vi "gyro-sweeper-V2.vi"() -> ()   [LabVIEW 2017]
uses:
  lorentzian.ctl
  circle corners.ctl
  peak -- parameters -- complex fit.ctl
  wavepacket.ctl
  filter method control.ctl
  cursor winow.ctl
  parameters -- scan monitor control.ctl
  freq scan type.ctl
  filename-pattern.ctl
  show-win- control.ctl
  PLL data source.ctl
  plot refs -- filter related.ctl
  cursor window action.ctl
  data source action.ctl
  publisher action.ctl
  file -- read-write control.ctl
  KM_file -- read-write control.ctl
  filename-action.ctl
  agregator -- action.ctl
  cursor action.ctl
  2Dwindow.ctl
  <vilib>/Analysis/baseanly.llb/A x B.vi
  <vilib>/Analysis/baseanly.llb/Complex A x B.vi
  line -- complex.vi
  Q -- check range -- i -- integer.vi
  Q - not nan -- real.vi
  linear interpolation - real.vi
  filter - complex - four.vi
  peak -- PM find lorenzian - V3.vi
  array -- sort 2D array -- Complex.vi/05c44075-957c-bc42-b6fa-2799d0bc0485.vi
  Q - not nan -- integer.vi
  tale of three indices.vi
  filter -- window span logic.vi
  linear interp iiii- complex - z-omega - divide.vi
  linear interpolation iiii- complex.vi
  containing bix.vi
  peak -- guess at omega -- dzdomega V2.vi
  <vilib>/Array/Sort 2D Array - Pop Stack.vi
  <vilib>/Array/Sort 2D Array - Push Stack.vi
  command stack.vi
  tale of three indices -- check state.vi
  peak -- z center from mult phase points.vi
  peak -- estimate for lorentzian.vi
  peak -- fake phase around center.vi
  peak -- get weights.vi
  peak -- four corner circle transformation logic.vi
  peak - fit phase around center - V2.vi
  circle center from three points.vi
  <vilib>/Utility/error.llb/Clear Errors.vi
  <vilib>/Analysis/Matrix/Numeric/Conversions/Array To Matrix.vi
  <vilib>/Analysis/Matrix/Numeric/Conversions/Array To Matrix - RA2.vi
  <vilib>/Analysis/baseanly.llb/Inverse Matrix.vi
  <vilib>/Analysis/baseanly.llb/Real Inverse Matrix.vi
  peak -- fit function -- minus arctan.vi
  <vilib>/gmath/NumericalOptimization/Nonlinear Curve Fit.vi
  <vilib>/gmath/NumericalOptimization/Nonlinear Curve Fit LM.vi
  KM_filter pipe - plot staff - more - V3.vi
panel:
  in  "all":enum32{"all"}(tab)
  in  "subtract bgnd !":bool
  out "Plot: circle sweep window":cluster{"all rows":dbl[], "all rows":dbl[]}[](graph)
  in  "sweeper panel":enum32{"circles sweep", "other"}(tab)
  in  "history length":i64=5
  out "fit is fine":bool=TRUE
  in  "gamma factor":dbl=1.6
  in  "Auto-update sweep window!":bool
  in  "scan type":T1
  in  "N":i64=257
  in  "sweep! :r":bool
  in  "delay-circle(msec)":i64
  out "scan progress":i32(slide)=256 min=0 max=257 scale=0.0..257.0
  out "circle frequency (Hz)":dbl=44934.75723893914 format="%#11_11f"
  out "circle gamma (Hz)":dbl=11.158120659005691 format="%#11_11f"
  out "circle phase (rad)":dbl=-1.4840328638382214 format="%#11_11f"
  out "circle Q":dbl=4027.0900998612533 format="%#11_11f"
  in  "beep!":bool
  in  "save data":enum32{"save/read"}(tab)
  in  "freqsweep name template":T2={"prefix"="lsco0.2", "group"="f"}
  in  "Save folder":path=path "/Users/arkady/Desktop/local_data/TaAs-quirk-Jan2018-losalamos"
  in  "freq sweep file name":string="f010_lsco0.2_012518.dat"
  in  "read from disk :l":bool
  in  "read file":path=path "/Users/arkady/Desktop/local_data/TaAs-quirk-Jan2018-losalamos/9w/f006_rucl3_012518.dat"
  in  "win":T3={"cen (Hz)"=44935.274309827895, "win (Hz)"=39.462177081403425, "left (Hz)"=44915.5432212872, "right (Hz)"=44955.005398368594}
  in  "PLL data source":T4=enum."MFLI"
  in  "Tab : everything":enum32{"Everything", "even more "}(tab)
  in  "Tab :  Fit controls":enum32{"complex plane", "complex plane 2"}(tab)
  in  "Plot: fragment - filter":cluster{dbl[], dbl[]}[](graph)=[{array[255 elements], array[255 elements]}, {array[255 elements], array[255 elements]}, {array[255 elements], array[255 elements]}, {array[255 elements], array[255 elements]}]
  in  "scale gauge: Plot: complex plane - filter":dbl(slide)=9.999999999999991e-05 min=0.0 max=0.3 step=1e-05 scale=0.0001..0.3 scale format="%#_5g"
  in  "Plot: complex plane - filter":cluster{dbl[], dbl[]}[](graph)=[{array[255 elements], array[255 elements]}, {array[255 elements], array[255 elements]}, {[-8.455997466784519e-05, -8.536551810596276e-05, -8.777896930838301e-05, -9.1790803485811e-05, -9.73851877615811e-05, -0.00010454004365678785, -0.00011322713422395566, -0.00012341217548537004, -0.00013505497173627495, -0.00014810957417895574, -0.00016252446226165164, -0.0001782427470066363, -0.00019520239552502235, -0.00021333647583223424, -0.00023257342099797256, -0.00025283731158819243, -0.00027404817528442526, -0.0002961223024979839, -0.0003189725767334659, -0.0003425088183977611, -0.0003666381406977065, -0.000391265316221823, -0.00041629315275940325, -0.00044162287687376416, -0.00046715452371587666, -0.000492787331539955, -0.000518420139364033, -0.0005439517862061456, -0.0005692815103205066, -0.0005943093468580867, -0.0006189365223822033, -0.0006430658446821486, -0.0006666020863464437, -0.0006894523605819259, -0.0007115264877954845, -0.0007327373514917173, -0.0007530012420819372, -0.0007722381872476754, -0.0007903722675548874, -0.0008073319160732736, -0.0008230502008182579, -0.000837465088900954, -0.0008505196913436348, -0.0008621624875945397, -0.0008723475288559541, -0.0008810346194231219, -0.0008881894753183286, -0.0008937838595940987, -0.0008977956937715266, -0.0009002091449739469, -0.0009010146884120644, -0.0009002091449739469, -0.0008977956937715266, -0.0008937838595940986, -0.0008881894753183286, -0.0008810346194231219, -0.000872347528855954, -0.0008621624875945397, -0.0008505196913436348, -0.000837465088900954, -0.0008230502008182579, -0.0008073319160732733, -0.0007903722675548873, -0.0007722381872476754, -0.0007530012420819371, -0.0007327373514917174, -0.0007115264877954843, -0.0006894523605819258, -0.0006666020863464435, -0.0006430658446821485, -0.0006189365223822033, -0.0005943093468580865, -0.0005692815103205065, -0.0005439517862061453, -0.0005184201393640329, -0.000492787331539955, -0.0004671545237158765, -0.00044162287687376416, -0.000416293152759403, -0.00039126531622182294, -0.00036663814069770655, -0.00034250881839776096, -0.00031897257673346594, -0.0002961223024979837, -0.0002740481752844252, -0.0002528373115881922, -0.0002325734209979724, -0.00021333647583223424, -0.0001952023955250222, -0.0001782427470066362, -0.00016252446226165153, -0.00014810957417895563, -0.00013505497173627495, -0.00012341217548536993, -0.0001132271342239556, -0.00010454004365678774, -9.738518776158104e-05, -9.1790803485811e-05, -8.777896930838301e-05, -8.536551810596276e-05], [0.004141207599747948, 0.004166840407572026, 0.004192372054414139, 0.0042177017785285, 0.00424272961506608, 0.0042673567905901965, 0.004291486112890142, 0.004315022354554437, 0.004337872628789919, 0.004359946756003478, 0.004381157619699711, 0.004401421510289931, 0.004420658455455669, 0.004438792535762881, 0.004455752184281267, 0.004471470469026252, 0.004485885357108948, 0.004498939959551629, 0.004510582755802533, 0.004520767797063948, 0.004529454887631116, 0.004536609743526323, 0.004542204127802092, 0.0045462159619795205, 0.00454862941318194, 0.004549434956620058, 0.00454862941318194, 0.0045462159619795205, 0.004542204127802092, 0.004536609743526323, 0.004529454887631116, 0.004520767797063948, 0.004510582755802533, 0.004498939959551629, 0.004485885357108948, 0.004471470469026252, 0.004455752184281267, 0.004438792535762881, 0.004420658455455669, 0.004401421510289931, 0.004381157619699711, 0.004359946756003478, 0.004337872628789919, 0.004315022354554437, 0.004291486112890142, 0.0042673567905901965, 0.00424272961506608, 0.0042177017785285, 0.004192372054414139, 0.004166840407572026, 0.004141207599747948, 0.0041155747919238705, 0.004090043145081758, 0.0040647134209673965, 0.0040396855844298165, 0.0040150584089057, 0.0039909290866057545, 0.00396739284494146, 0.003944542570705978, 0.003922468443492419, 0.003901257579796186, 0.003880993689205966, 0.003861756744040228, 0.003843622663733016, 0.0038266630152146296, 0.0038109447304696454, 0.003796529842386949, 0.0037834752399442686, 0.0037718324436933634, 0.0037616474024319492, 0.0037529603118647815, 0.0037458054559695747, 0.0037402110716938048, 0.0037361992375163767, 0.0037337857863139565, 0.0037329802428758387, 0.0037337857863139565, 0.0037361992375163767, 0.0037402110716938048, 0.0037458054559695747, 0.0037529603118647815, 0.0037616474024319492, 0.0037718324436933634, 0.0037834752399442686, 0.003796529842386949, 0.0038109447304696454, 0.00382666301521463, 0.003843622663733016, 0.003861756744040228, 0.0038809936892059663, 0.0039012575797961863, 0.003922468443492419, 0.003944542570705978, 0.00396739284494146, 0.0039909290866057545, 0.0040150584089057, 0.0040396855844298165, 0.0040647134209673965, 0.004090043145081758, 0.0041155747919238705]}, {[0.00016018653422290237, -9.655871916433519e-05, 0.00023322284291397248], [-0.00028197255148921553, -1.017876794960279e-06, -0.00018735204694998037]}, {[0.00016865843187043812, 0.00017215317328655273, 0.00017564791470266734, 0.00017914265611878197, 0.00018263739753489658, 0.0001861321389510112, 0.0001896268803671258, 0.0001931216217832404, 0.00019661636319935505, 0.00020011110461546966, 0.00020360584603158427, 0.00020710058744769888, 0.0002105953288638135, 0.00021409007027992812, 0.00021758481169604273, 0.00022107955311215734, 0.00022457429452827195, 0.0002280690359443866, 0.00023156377736050117, 0.0002350585187766158], [-0.00027606938786554, -0.00027143787714636365, -0.00026680636642718733, -0.00026217485570801096, -0.00025754334498883464, -0.00025291183426965827, -0.00024828032355048195, -0.00024364881283130558, -0.00023901730211212924, -0.0002343857913929529, -0.00022975428067377655, -0.0002251227699546002, -0.00022049125923542386, -0.00021585974851624751, -0.00021122823779707114, -0.00020659672707789482, -0.00020196521635871845, -0.00019733370563954213, -0.00019270219492036576, -0.00018807068420118942]}, {[-9.655871916433519e-05, -9.088660415427566e-05, -8.521448914421613e-05, -7.95423741341566e-05, -7.387025912409707e-05, -6.819814411403754e-05, -6.252602910397802e-05, -5.685391409391849e-05, -5.118179908385896e-05, -4.550968407379943e-05, -3.98375690637399e-05, -3.416545405368038e-05, -2.8493339043620856e-05, -2.282122403356132e-05, -1.7149109023501796e-05, -1.147699401344226e-05, -5.804879003382736e-06, -1.3276399332321333e-07, 5.539351016736323e-06, 1.1211466026795846e-05], [-1.017876794960279e-06, -1.017876794960279e-06, -1.017876794960279e-06, -1.017876794960279e-06, -1.017876794960279e-06, -1.017876794960279e-06, -1.017876794960279e-06, -1.017876794960279e-06, -1.017876794960279e-06, -1.017876794960279e-06, -1.017876794960279e-06, -1.017876794960279e-06, -1.017876794960279e-06, -1.017876794960279e-06, -1.017876794960279e-06, -1.017876794960279e-06, -1.017876794960279e-06, -1.017876794960279e-06, -1.017876794960279e-06, -1.017876794960279e-06]}]
  out "Plot: dz/domega":cluster{"omega out":dbl[], dbl[]}(graph)
  out "Plot: win omega":T5(graph)
  out "Plot: phase":cluster{"omega out":dbl[], dbl[]}(graph)
  out "Plot: phase around center":cluster{dbl[], dbl[]}[](graph)
  out "Plot: fragment":cluster{dbl[], dbl[]}[](graph)
  out "Plot: complex plane":cluster{dbl[], dbl[]}[](graph)=[{array[255 elements], array[255 elements]}, {[-0.00010617557464667055, -0.00010929113388811687, -0.00011858867738207354, -0.00013392157731355743, -0.00015504802469121866, -0.0001816348428195835, -0.0002132627416945725, -0.000249432930457336, -0.0002895749836240618, -0.00033305583703661034, -0.0003791897716624629, -0.00042724922779349337, -0.0004764762790971875, -0.0005260945855676712, -0.0005753216368713655, -0.0006233810930023958, -0.0006695150276282485, -0.0007129958810407971, -0.0007531379342075228, -0.0007893081229702864, -0.0008209360218452751, -0.0008475228399736401, -0.0008686492873513014, -0.0008839821872827852, -0.0008932797307767419, -0.0008963952900181882, -0.0008932797307767419, -0.0008839821872827852, -0.0008686492873513013, -0.0008475228399736401, -0.0008209360218452751, -0.0007893081229702863, -0.0007531379342075226, -0.0007129958810407969, -0.0006695150276282483, -0.0006233810930023958, -0.0005753216368713655, -0.0005260945855676711, -0.00047647627909718735, -0.0004272492277934931, -0.00037918977166246303, -0.00033305583703661034, -0.00028957498362406167, -0.00024943293045733586, -0.00021326274169457238, -0.0001816348428195834, -0.00015504802469121866, -0.00013392157731355737, -0.00011858867738207348, -0.00010929113388811687], [0.004141386571247566, 0.004190906967324454, 0.0042396463971731595, 0.004286836210869443, 0.004331732196861486, 0.004373626318630633, 0.004411857880850249, 0.0044458239489457005, 0.004474988857732779, 0.0044988926591776396, 0.004517158376052058, 0.004529497947089514, 0.004535716769883444, 0.004535716769883444, 0.004529497947089514, 0.004517158376052058, 0.0044988926591776396, 0.004474988857732779, 0.0044458239489457005, 0.004411857880850249, 0.004373626318630633, 0.004331732196861486, 0.004286836210869443, 0.0042396463971731595, 0.004190906967324454, 0.004141386571247566, 0.004091866175170678, 0.004043126745321973, 0.003995936931625689, 0.003951040945633646, 0.003909146823864499, 0.0038709152616448837, 0.0038369491935494313, 0.003807784284762353, 0.0037838804833174922, 0.0037656147664430744, 0.0037532751954056187, 0.0037470563726116884, 0.0037470563726116884, 0.0037532751954056187, 0.0037656147664430744, 0.0037838804833174927, 0.003807784284762353, 0.0038369491935494318, 0.003870915261644884, 0.0039091468238645, 0.003951040945633646, 0.003995936931625689, 0.004043126745321973, 0.004091866175170678]}, {[-0.00010766181539318114, -0.00014702417708710596, -0.00018638653878103078, -0.00022574890047495562, -0.0002651112621688804, -0.00030447362386280526, -0.0003438359855567301, -0.0003831983472506549, -0.00042256070894457974, -0.0004619230706385046, -0.0005012854323324294, -0.0005406477940263542, -0.0005800101557202791, -0.0006193725174142039, -0.0006587348791081286, -0.0006980972408020535, -0.0007374596024959783, -0.0007768219641899032, -0.000816184325883828, -0.0008555466875777528], [0.004175624676161894, 0.004172200865670462, 0.004168777055179028, 0.004165353244687596, 0.0041619294341961625, 0.00415850562370473, 0.004155081813213298, 0.004151658002721864, 0.004148234192230432, 0.0041448103817389986, 0.004141386571247566, 0.004137962760756134, 0.0041345389502647, 0.004131115139773268, 0.004127691329281835, 0.004124267518790402, 0.00412084370829897, 0.004117419897807536, 0.004113996087316104, 0.004110572276824671]}, {[-0.0004670473274181016, -0.00047047113790953435, -0.0004738949484009671, -0.0004773187588923999, -0.0004807425693838327, -0.0004841663798752655, -0.00048759019036669825, -0.0004910140008581311, -0.0004944378113495638, -0.0004978616218409966, -0.0005012854323324294, -0.0005047092428238621, -0.0005081330533152949, -0.0005115568638067277, -0.0005149806742981604, -0.0005184044847895932, -0.000521828295281026, -0.0005252521057724587, -0.0005286759162638915, -0.0005320997267553243], [0.0037477629543083172, 0.0037871253160022423, 0.003826487677696167, 0.003865850039390092, 0.0039052124010840166, 0.003944574762777942, 0.003983937124471867, 0.004023299486165791, 0.004062661847859716, 0.004102024209553641, 0.004141386571247566, 0.004180748932941491, 0.004220111294635415, 0.0042594736563293404, 0.0042988360180232655, 0.0043381983797171906, 0.004377560741411115, 0.00441692310310504, 0.004456285464798965, 0.00449564782649289]}, {[-0.1345621971793873, -0.13512978580258067, -0.13561317033829676, -0.13601204868693562, -0.13632617156251337, -0.13655534264845795, -0.13669941872030045, -0.13675830973518588, -0.1367319788881469, -0.1366204426351058, -0.1364237706825901, -0.1361420859441681, -0.1357755644636322, -0.13532443530497684, -0.13478898040924134, -0.1341695344183057, -0.13346648446575046, -0.13268026993491067, -0.13181138218427568, -0.1308603642404062], [0.028525297489512894, 0.02516387834181004, 0.021789321345350735, 0.01840373548841113, 0.015009236651946362, 0.01160794628723345, 0.008201990090033556, 0.004793496672101276, 0.0013845962308715039, -0.00202258078184437, -0.00542590499132186, -0.008823249430713024, -0.01221249087033164, -0.015591511144602398, -0.0189581984758458, -0.022310448794070212, -0.02564616705194721, -0.028963268534148004, -0.0322596801602224, -0.03553334178020699]}, {[-0.14932045372175862, -0.14995047709350323, -0.15048703392814808, -0.15092978889513722, -0.15127846528702854, -0.15153284519242702, -0.15169276963217218, -0.151758138658695, -0.15172891141848174, -0.15160510617760614, -0.15138680031031368, -0.1510741302506653, -0.15066729140727042, -0.15016653804116298, -0.14957218310689657, -0.14888459805695803, -0.1481042126096217, -0.1472315144803895, -0.1462670490771847, -0.1452114191594896], [0.031207435410939594, 0.027476260156989427, 0.023730501890919596, 0.019972501589716637, 0.016204607881240743, 0.012429175576409409, 0.008648564197517528, 0.004865136503612697, 0.0010812570138476487, -0.002700709470266971, -0.0064783993427869856, -0.01024945167051118, -0.014011509668487843, -0.017762222172928385, -0.02149924511060856, -0.02522024296383766, -0.028922890230081127, -0.03260487287532401, -0.03626388978026658, -0.03989765417844949]}, {array[255 elements], array[255 elements]}]
  in  "scale gauge: Plot: complex plane":dbl(slide)=9.999999999999991e-05 min=0.0 max=0.3 step=1e-05 scale=0.0001..1.0 scale format="%#_2g"
  out "window width (kHz)":dbl=76.27809365793496
  out "window center (kHz)":dbl=3399.029286744401
  out "# of points in window":dbl=953.475933538175
  in  "use fast fit!":bool
  out "lorentzian":T6={"Amplitude"=0.004408683465620264, "omega(0)"=44934.75723893914, "Gamma"=11.158120659005691, "phase"=-1.4840328638382214, "Q"=4027.0900998612533, "Norm  Ampl"=nan, "z (inf)"=-0.00010766181539318109+0.004175624676161894i, "4corners"={"z (-pi/2)"=-0.00046704732741810164+0.0037477629543083177i, "z(inf)"=-0.00010766181539318109+0.004175624676161894i, "z (pi/2)"=-0.0005355235372467572+0.004535010188186815i, "z center"=-0.0005012854323324294+0.004141386571247566i, "z(0)"=-0.0008949090492716776+0.004107148466333238i, "radius"=0.00039510985768575883}} {"z (inf)" format="%#9_9f"; "Q" format="%#9_9f"; "phase" format="%#9_9f"; "Gamma" format="%#9_9f"; "omega(0)" format="%#9_9f"}
  in  "plot staff!":enum16{"plot", "do not plot", "a"}(ring)
  in  "fit!":bool=TRUE
  in  "scan monitor control":T8={"gamma acc. frac. - min "=0.3, "gamma acc frac.. - max"=3.0, "peak acc. fraction (af)"=5.0, "min peak acc. window (kHz)"=0.5, "use"=enum."fraction", "abs gamma min(kHz)"=0.005, "abs gamma max(kHz)"=5.0, "# points"=5, "gamma-factor (fa)"=3.0, "interpolate"=enum."line", "init"=TRUE, "Unique strike parameters"=TRUE, "max peak acc. window (kHz)"=10.0, "spacing factor"=1.5, "iterate #"=1, "overwrite ctl?"=FALSE, "write _m files?"=FALSE, "max slope (kHz/sweep)"=0.5, "funnel state"=enum."funnel open"}
  in  "parameters: complex fit":T9={"main VI path"=path "", "scale factor"=3.0, "# of grid points"=200, "parameters: wavepacket"={"R"=0.5, "wave number"=22.0, "delta k"=7.0, "radii vector"=[], "radial section"=[], "wave vector"=22.0, "wavepacket is"=TRUE}, "span"=0.27789, "interference ?"=enum."cp z center", "filter method"=enum."three"} {"span" min=0.0 max=0.5 step=1e-05 scale=0.0001..0.5 scale format="%#_5f"; "parameters: wavepacket"."delta k" format="%#_3f"; "parameters: wavepacket"."wave number" format="%#_3f"; "parameters: wavepacket"."R" format="%#_3f"}
  in  "cursor bracket: circle window":T12={"left"=44915.5432212872, "right "=44955.005398368594, "center"=44935.274309827895, "window"=39.462177081403425, "cursors"=[0, 1, 2], "relative"=0, "absolute"=0, "fixed vertical offset"=0.0, "vertical offset"=0.0, "skew"=0.0, "default window frac"=0.1, "kind"=enum."symmetric", "skew.left"=0.5, "skew.right"=0.5, "Plot ref"=refnum, "wing order"=enum."forw"}
  in  "cursor bracket: fit boundaries":T12={"left"=45113.93683640631, "right "=45686.175933405, "center"=45400.056384905656, "window"=572.2390969986809, "cursors"=[3, 4, 5], "relative"=0, "absolute"=0, "fixed vertical offset"=0.0, "vertical offset"=0.0, "skew"=0.0, "default window frac"=0.1, "kind"=enum."symmetric", "skew.left"=0.5, "skew.right"=0.5, "Plot ref"=refnum, "wing order"=enum."forw"}
  # "three strikes"
  # "search window"
  # "linear extrapolation"
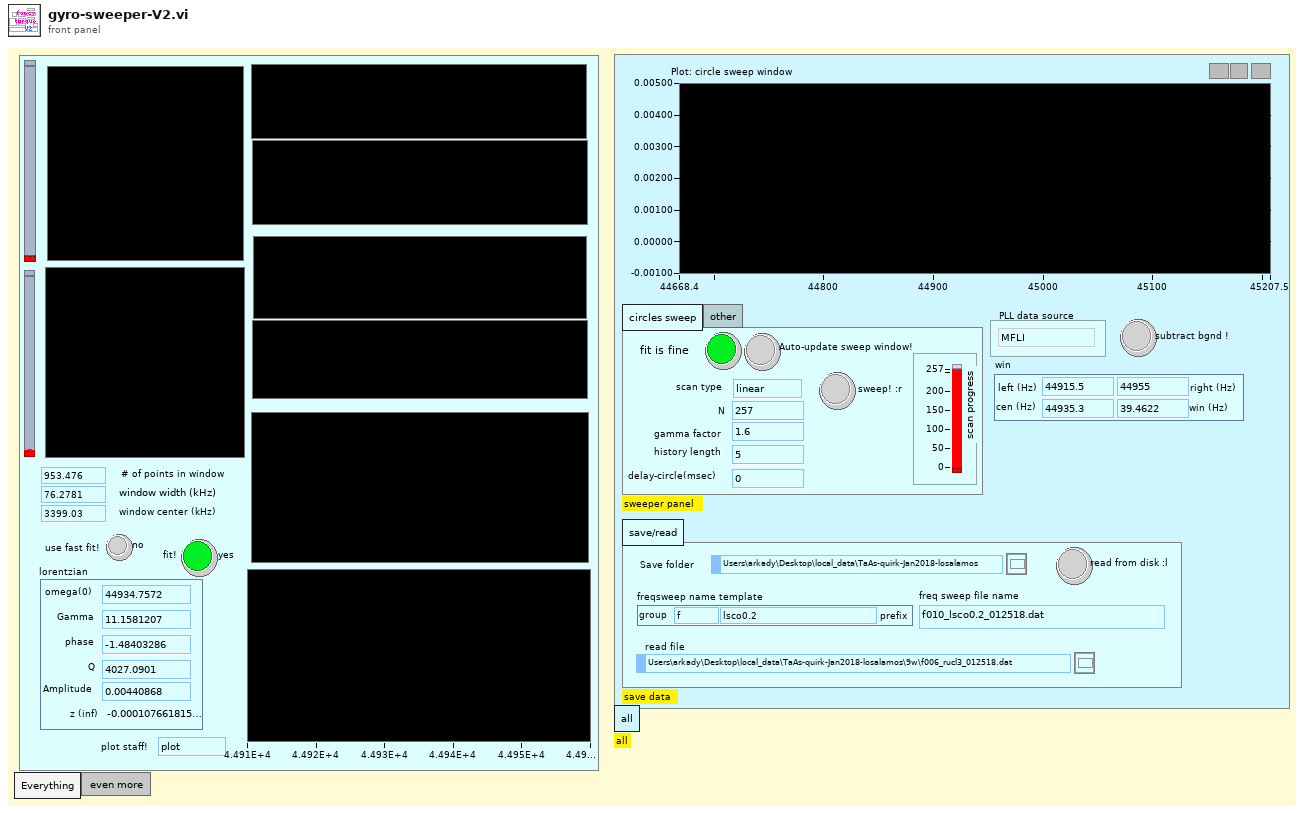
[diagram p1: front panel]
types:
  T1 = typedef "freq scan type.ctl" = enum16{"linear", "arctan"}
  T2 = typedef "filename-pattern.ctl" = cluster{"prefix":string, "group":string}
  T3 = typedef "show-win- control.ctl" = cluster{"cen (Hz)":dbl, "win (Hz)":dbl, "left (Hz)":dbl, "right (Hz)":dbl}
  T4 = typedef "PLL data source.ctl" = enum16{"meta", "MFLI"}
  T5 = cluster{"omega out":dbl[], "win omega out":dbl[]}
  T6 = typedef "lorentzian.ctl" = cluster{"Amplitude":dbl, "omega(0)":dbl, "Gamma":dbl, "phase":dbl, "Q":dbl, "Norm  Ampl":dbl, "z (inf)":cdb, "4corners":T7}
  T7 = typedef "circle corners.ctl" = cluster{"z (-pi/2)":cdb, "z(inf)":cdb, "z (pi/2)":cdb, "z center":cdb, "z(0)":cdb, "radius":dbl}
  T8 = typedef "parameters -- scan monitor control.ctl" = cluster{"gamma acc. frac. - min ":dbl, "gamma acc frac.. - max":dbl, "peak acc. fraction (af)":dbl, "min peak acc. window (kHz)":dbl, "use":enum16{"window", "fraction"}, "abs gamma min(kHz)":dbl, "abs gamma max(kHz)":dbl, "# points":i32, "gamma-factor (fa)":dbl, "interpolate":enum16{"line", "last"}, "init":bool, "Unique strike parameters":bool, "max peak acc. window (kHz)":dbl, "spacing factor":dbl, "iterate #":i32, "overwrite ctl?":bool, "write _m files?":bool, "max slope (kHz/sweep)":dbl, "funnel state":enum16{"funnel open", "funnel closed"}}
  T9 = typedef "peak -- parameters -- complex fit.ctl" = cluster{"main VI path":path, "scale factor":dbl, "# of grid points":i32, "parameters: wavepacket":T10, "span":dbl, "interference ?":enum16{"cp z center", "pm zcenter", "fancy"}, "filter method":T11}
  T10 = typedef "wavepacket.ctl" = cluster{"R":dbl, "wave number":dbl, "delta k":dbl, "radii vector":dbl[], "radial section":cdb[], "wave vector":dbl, "wavepacket is":bool}
  T11 = typedef "filter method control.ctl" = enum16{"four", "five", "one", "two", "three", "zero", "minus one", "minus two"}
  T12 = typedef "cursor winow.ctl" = cluster{"left":dbl, "right ":dbl, "center":dbl, "window":dbl, "cursors":i32[], "relative":i32, "absolute":i32, "fixed vertical offset":dbl, "vertical offset":dbl, "skew":dbl, "default window frac":dbl, "kind":enum16{"symmetric", "skewed", "fancy"}, "skew.left":dbl, "skew.right":dbl, "Plot ref":refnum<vi>, "wing order":enum16{"forw", "back"}}
  T13 = typedef "data source action.ctl" = enum16{"set", "get", "init"}
  T14 = typedef "cursor window action.ctl" = enum16{"balance", "h. offset change", "cursor moves", "change center", "change window", "init", "check", "reset", "set y to middle", "idle", "-write all Y", "-write left.X", "-write center.X", "-write right.X", "-write all X", "-change center", "-change window", "-change skew", "-read cursor 2", "-read cursor 1", "-read cursor 0", "-read all cursors", "-reset", "-read plot scale", "-set y to middle", "-Q: center.Y is visible", "-Q: window is visible", "-parse center.Y", "-right left from center", "-left move", "-right move", "-set center.Y", "-empty", "-set cursors to default", "-check", "-write center.Y", "-copy cursor 1", "-copy cursor 0", "-copy cursor 2", "move right", "move left", "shrink", "broaden", "skew up", "skew down", "-write plot scale", "zoom X", "change cen&win", "zoom to all data", "color--red", "color--green", "color--yellow", "read", "zoom out", "zoom in", "slide right", "slide left", "set range aspect ratio to 1"}
  T15 = typedef "plot refs -- filter related.ctl" = cluster{"Plot: complex plane - filter":refnum<vi>, "Plot: dz/domega":refnum<vi>, "Plot: fragment filter":refnum<vi>, "Plot: win omega":refnum<vi>, "Plot: phase":refnum<vi>, "Plot: phase around center":refnum<vi>, "Plot: complex plane":refnum<vi>, "Plot: fragment":refnum<vi>}
  T16 = typedef "publisher action.ctl" = enum16{"set", "get"}
  T17 = typedef "file -- read-write control.ctl" = enum16{"read", "write all", "append one line"}
  T18 = typedef "filename-action.ctl" = enum16{"rewrite", "parse", "force pattern", "uniquenum"}
  T19 = typedef "KM_file -- read-write control.ctl" = enum16{"read", "write all", "append one line"}
  T20 = typedef "agregator -- action.ctl" = enum16{"append", "interpolate", "empty!", "force", "init", "scale", "read last"}
  T21 = typedef "interpolation state - real.ctl" = cluster{"requested size":i32, "Array":dbl[], "actual number of elements":i32}
  T22 = typedef "2Dwindow.ctl" = cluster{"window y":dbl, "center x":dbl, "center y":dbl, "window x":dbl}
  T23 = typedef "cursor action.ctl" = enum16{"range", "read", "write", "check", "zoom out", "smart zoom out", "zoom to aspect ratio 1", "zoom to win", "zoom out 20%", "zoom in 20%"}
  T24 = typedef "eventvkey.ctl" = enum16{"ASCII", "Enter", "Return", "Shift", "Ctrl", "Alt", "Cmd", "Opt", "Caps", "NumLock", "Clear", "Break", "Up", "Down", "Left", "Right", "Insert", "Delete", "Home", "End", "PageUp", "PageDown", "Escape", "Help", "Pause", "ScrollLock", "F1", "F2", "F3", "F4", "F5", "F6", "F7", "F8", "F9", "F10", "F11", "F12", "F13", "F14", "F15", "F16", "F17", "F18", "F19", "F20", "F21", "F22", "F23", "F24", "Play", "VolumeUp", "VolumeDown", "Mute", "Two Byte Char"}
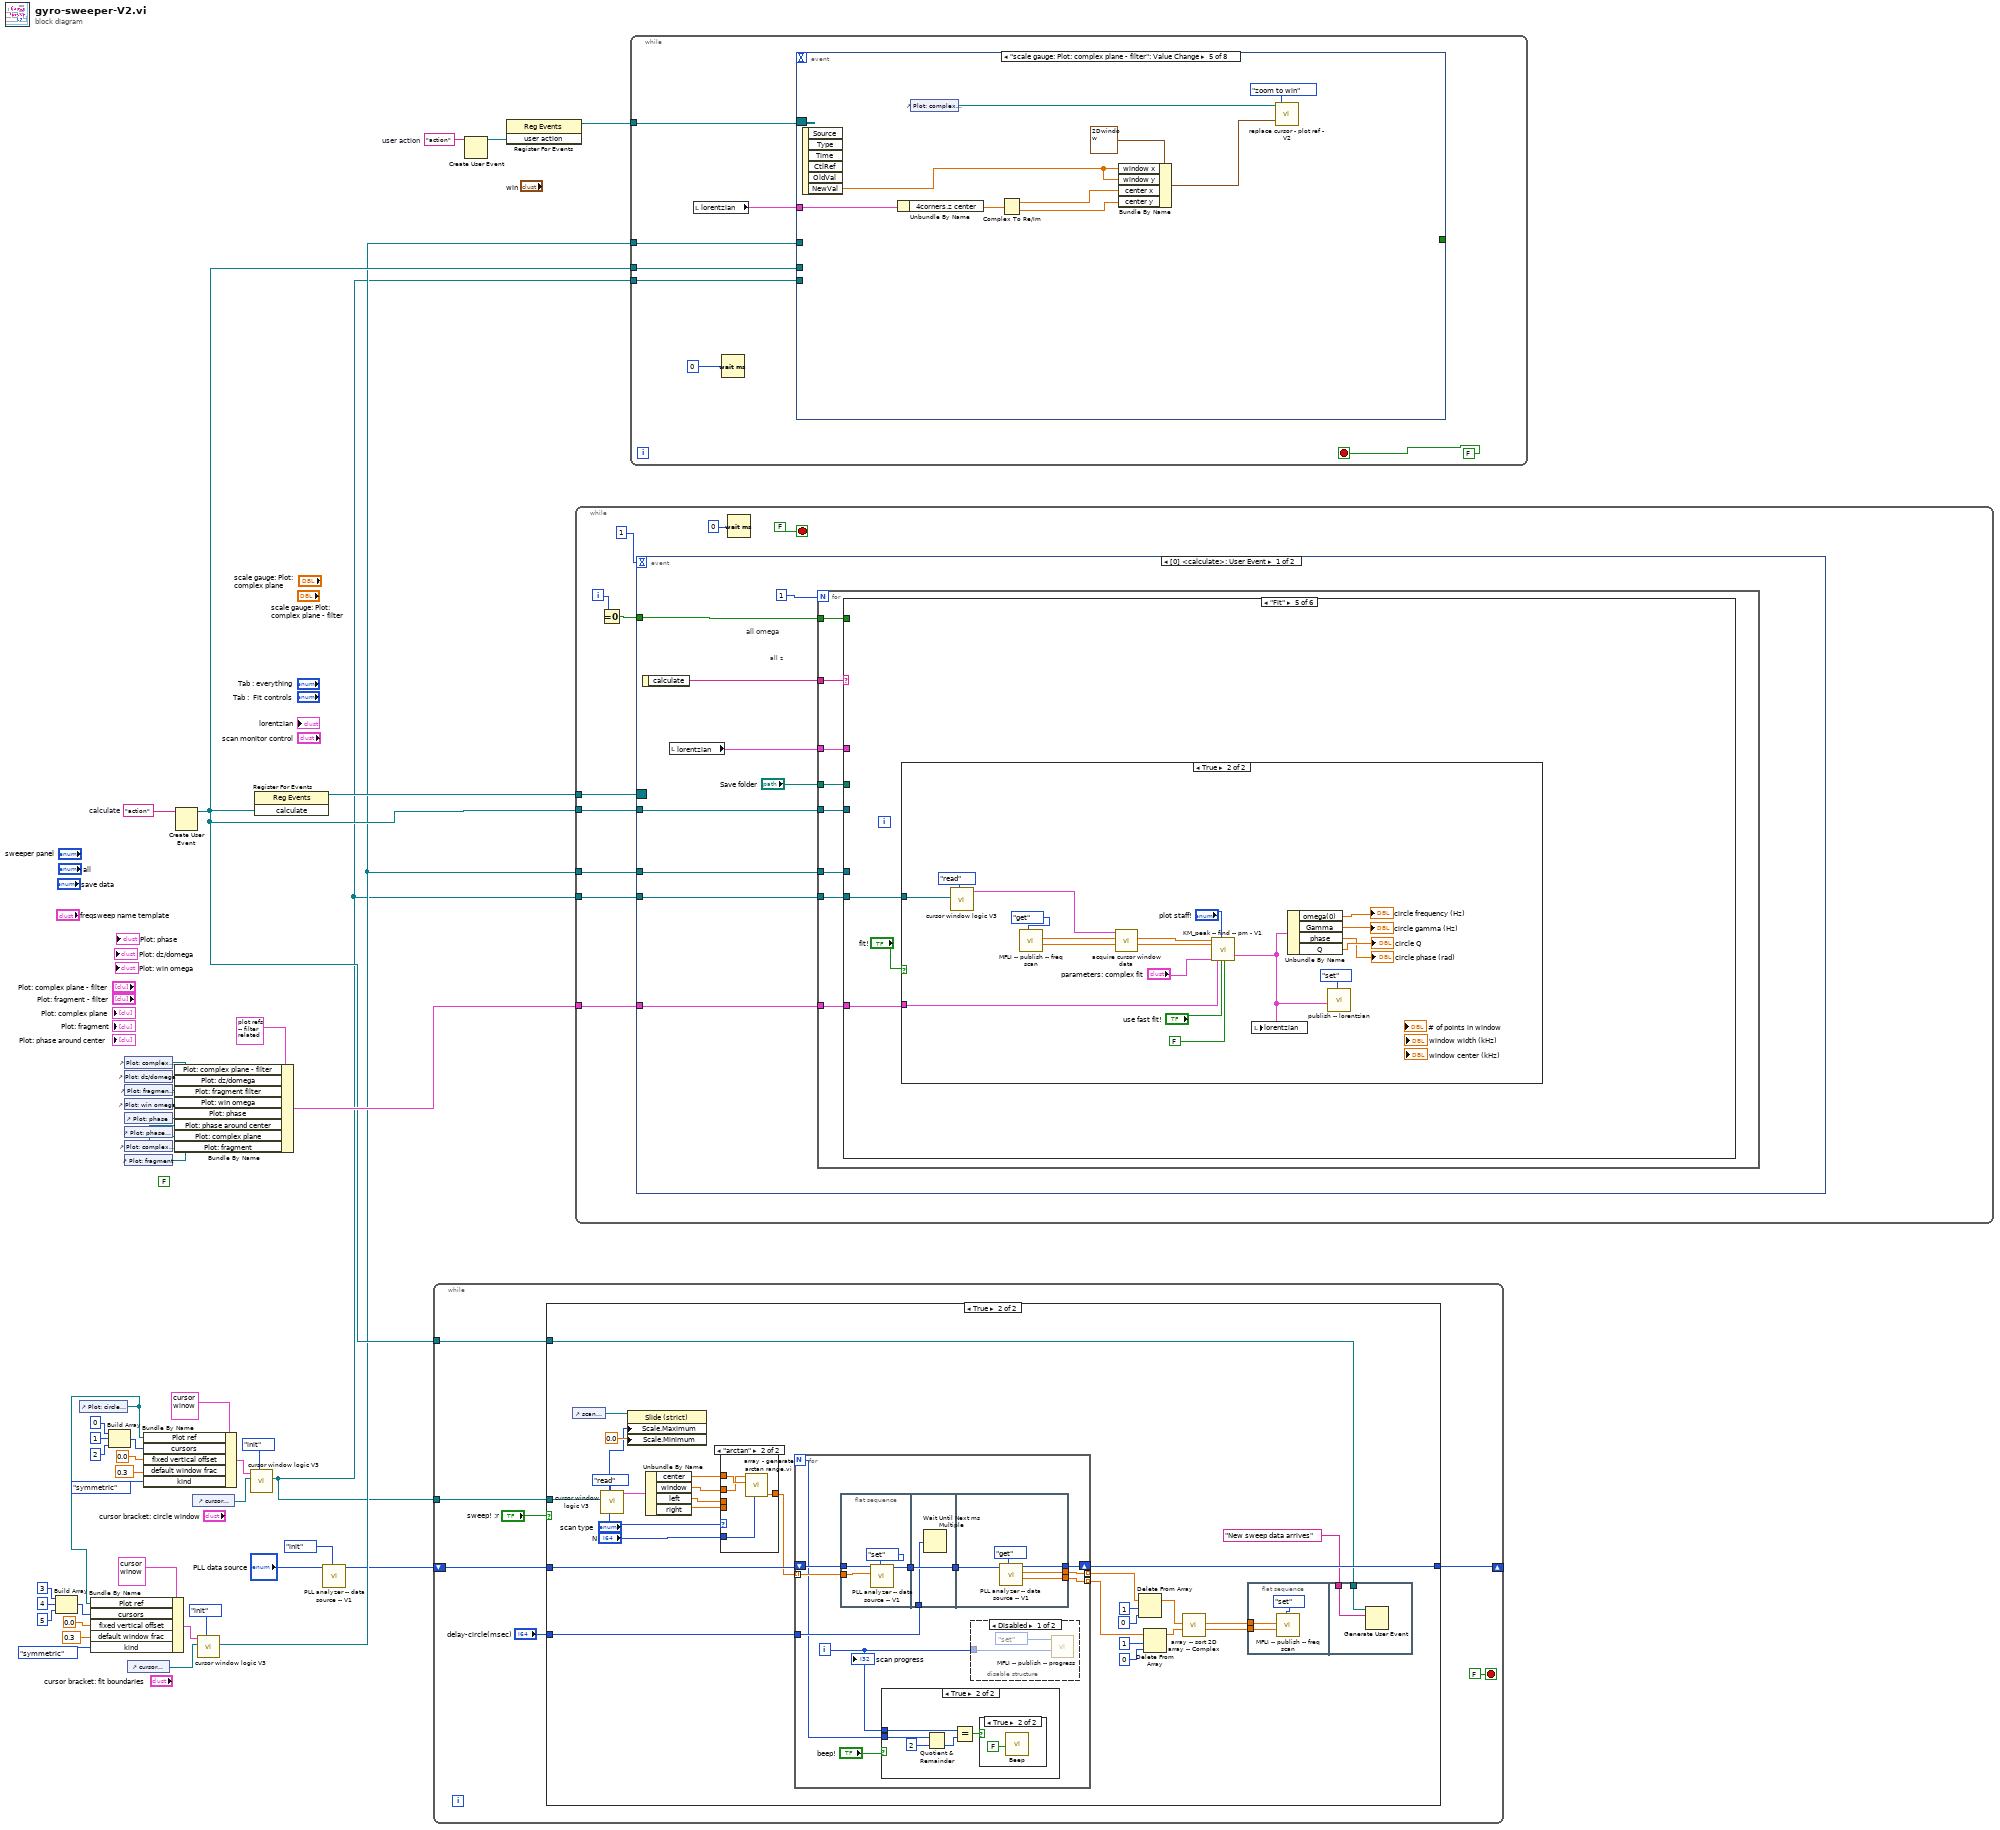
[diagram p0: block diagram]
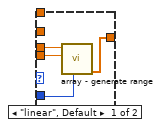
[diagram p6: hidden frame]
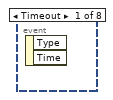
[diagram p7: hidden frame]
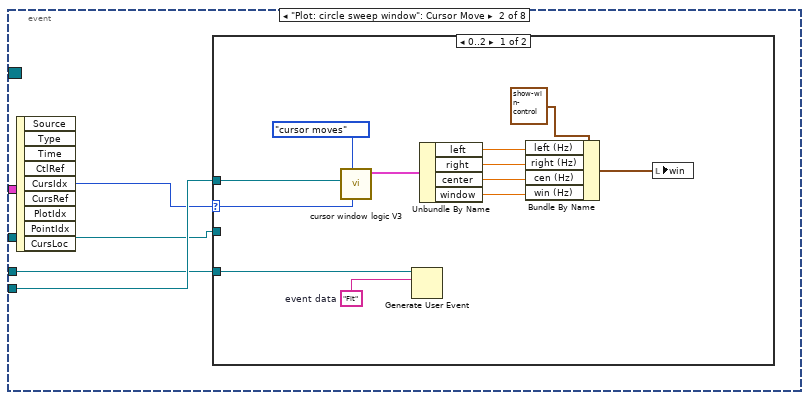
[diagram p8: hidden frame]
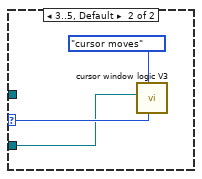
[diagram p9: hidden frame]
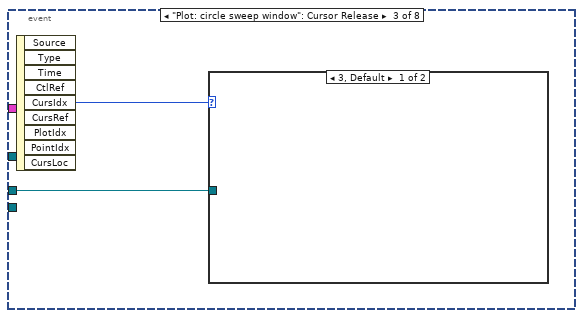
[diagram p10: hidden frame]
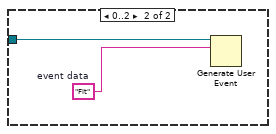
[diagram p11: hidden frame]
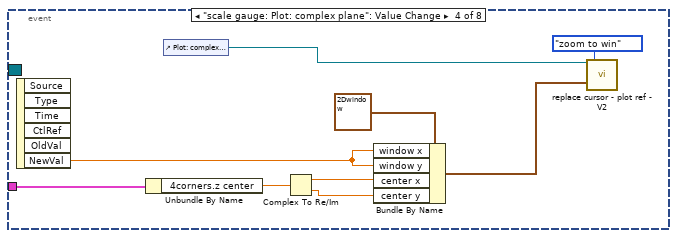
[diagram p12: hidden frame]
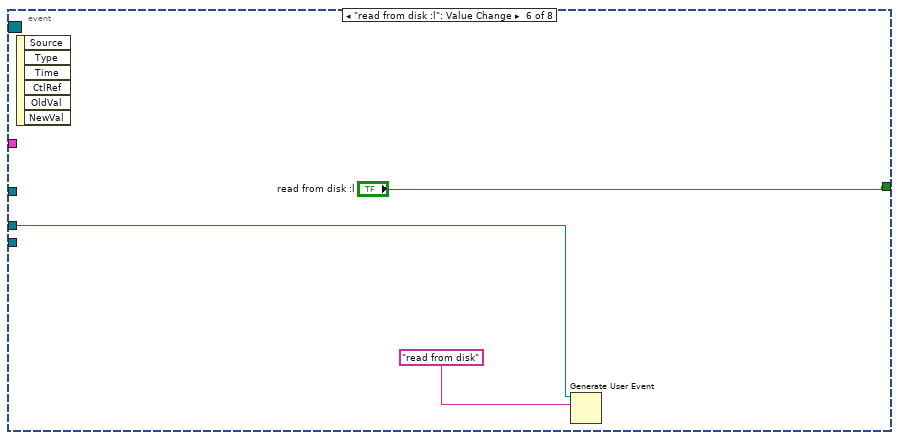
[diagram p13: hidden frame]
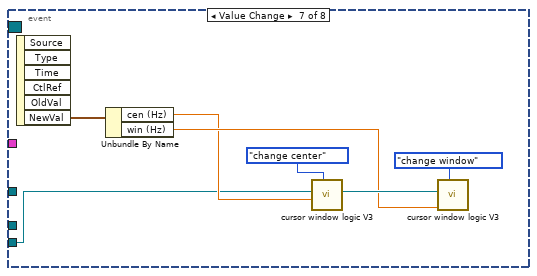
[diagram p14: hidden frame]
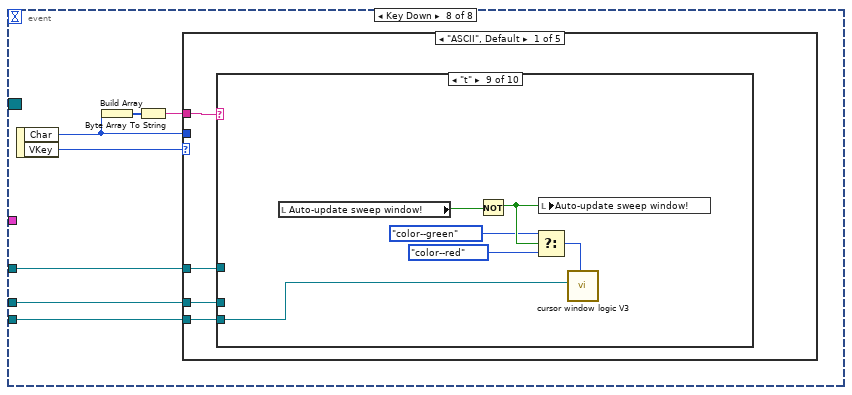
[diagram p15: hidden frame]
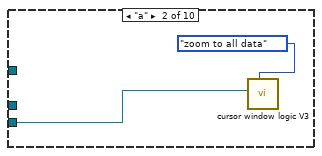
[diagram p17: hidden frame]
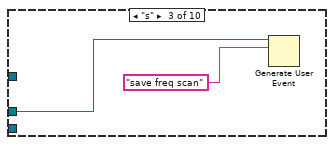
[diagram p18: hidden frame]
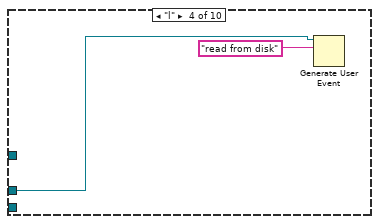
[diagram p19: hidden frame]
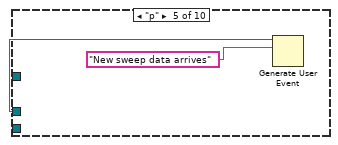
[diagram p20: hidden frame]
diagram:
  w41 = "action"  # user action
  w43 = "action"  # calculate
  (unwired) FALSE
  n1 = Build Array(3, 4, 5) -> (w17:i32[])
  n2 = control-ref of="Plot: circle sweep window"() -> (w6:refnum<vi>)
  n3 = Bundle By Name(cluster=T12 {"left"=0.0, "right "=0.0, "center"=0.0, "window"=0.0, "cursors"=[], "relative"=0, "absolute"=0, "fixed vertical offset"=0.0, "vertical offset"=0.0, "skew"=0.0, "default window frac"=0.0, "kind"=enum."symmetric", "skew.left"=0.0, "skew.right"=0.0, "Plot ref"=refnum, "wing order"=enum."forw"} ("cursor bracket: All, data window"), "Plot ref"=w6, "cursors"=w17, "fixed vertical offset"=0.0, "default window frac"=0.3 ("fixed vertical offset"), "kind"=enum16{"symmetric", "skewed", "fancy"}."symmetric") -> (w9:T12)
  n4 = Build Array(0, 1, 2) -> (w28:i32[])
  n5 = control-ref of="Plot: complex plane - filter"() -> (w38:refnum<vi>)
  n6 = control-ref of="Plot: dz/domega"() -> (w37:refnum<vi>)
  n7 = control-ref of="Plot: fragment - filter"() -> (w36:refnum<vi>)
  n8 = control-ref of="Plot: win omega"() -> (w35:refnum<vi>)
  n9 = control-ref of="Plot: phase"() -> (w34:refnum<vi>)
  n10 = control-ref of="Plot: phase around center"() -> (w32:refnum<vi>)
  n11 = control-ref of="Plot: complex plane"() -> (w31:refnum<vi>)
  n12 = control-ref of="Plot: fragment"() -> (w30:refnum<vi>)
  n13 = control-ref of="cursor bracket: fit boundaries"() -> (w7:refnum<vi>)
  n14 = Bundle By Name(cluster=T12 {"left"=0.0, "right "=0.0, "center"=0.0, "window"=0.0, "cursors"=[], "relative"=0, "absolute"=0, "fixed vertical offset"=0.0, "vertical offset"=0.0, "skew"=0.0, "default window frac"=0.0, "kind"=enum."symmetric", "skew.left"=0.0, "skew.right"=0.0, "Plot ref"=refnum, "wing order"=enum."forw"} ("cursor bracket: All, data window"), "Plot ref"=w6, "cursors"=w28, "fixed vertical offset"=0.0, "default window frac"=0.3 ("fixed vertical offset"), "kind"=enum16{"symmetric", "skewed", "fancy"}."symmetric") -> (w20:T12)
  n15 = Bundle By Name(cluster=T15 {"Plot: complex plane - filter"=refnum, "Plot: dz/domega"=refnum, "Plot: fragment filter"=refnum, "Plot: win omega"=refnum, "Plot: phase"=refnum, "Plot: phase around center"=refnum, "Plot: complex plane"=refnum, "Plot: fragment"=refnum} ("plots: filter related"), "Plot: complex plane - filter"=w38, "Plot: dz/domega"=w37, "Plot: fragment filter"=w36, "Plot: win omega"=w35, "Plot: phase"=w34, "Plot: phase around center"=w32, "Plot: complex plane"=w31, "Plot: fragment"=w30) -> (w33:T15)
  n16 = Create User Event(user event datatype=w43) -> (user event=w29:refnum<user-event>)  [unwired: 1 in, 1 out]
  n17 = control-ref of="cursor bracket: circle window"() -> (w19:refnum<vi>)
  n18 = call "cursor window logic V3.vi"("cursor window action"=cursor_window_action."init", "cursor window in"=w7, "cursor window init"=w9) -> ("cursor window out"=w5:refnum<vi>)  [unwired: 7 in, 1 out]
  n19 = call "cursor window logic V3.vi"("cursor window action"=cursor_window_action."init", "cursor window in"=w19, "cursor window init"=w20) -> ("cursor window out"=w4:refnum<vi>)  [unwired: 7 in, 1 out]
  n20 = register-events(w29) -> (reference out=w44:refnum<event-registration>)  [unwired: 2 in, 1 out]
  n21 = call "PLL analyzer -- data source -- V1.vi"("data source action"=data_source_action."init", "PLL data source"="PLL data source") -> ("PLL data source OUT"=w1:T4)  [unwired: 7 in, 2 out]
  n22 = while {
    tunnel: w29 -> [w51]
    tunnel: w4 -> [w49]
    shift-right: [w46] -> _
    shift-left: w1 -> [w45]
    stop <- FALSE stop-if-true
    n23 = case shown="True" "sweep! :r" {
      tunnel: w51 -> [_ w59]
      tunnel: w49 -> [_ w79]
      tunnel: "delay-circle(msec)" -> [_ w64]
      tunnel: [w52 w63] -> w46
      tunnel: w45 -> [w52 w62]
      frame False {
      }
      frame True {
        n24 = control-ref of="scan progress"() -> (w67:refnum<vi>)
        n25 = call "cursor window logic V3.vi"("cursor window action"=cursor_window_action."read", "cursor window in"=w79) -> ("cursor window out"=w69:T12)  [unwired: 8 in, 1 out]
        n26 = property class="Slide (strict)"(reference=w67, "Scale.Maximum"="N", "Scale.Minimum"=0.0 ("Data Entry Limits:Minimum")) -> ()  [unwired: 1 in, 2 out]
        n27 = Unbundle By Name(w69) -> ("center"=w73:dbl, "window"=w72:dbl, "left"=w71:dbl, "right"=w70:dbl)
        n28 = case shown="\"arctan\"" "scan type" {
          tunnel: [w113 w117] -> w53
          tunnel: w73 -> [_ w116]
          tunnel: w72 -> [_ w115]
          tunnel: w71 -> [w112 _]
          tunnel: w70 -> [w111 _]
          tunnel: "N" -> [w110 w114]
          frame "linear", Default {
            n29 = call "array - generate range.vi"("N"=w110, "freq max"=w111, "freq min"=w112) -> ("Array"=w113:dbl[])  [unwired: 7 in, 1 out]
          }
          frame "arctan" {
            n30 = call "array - generate arctan range.vi.vi"("N"=w114, "omega0"=w116, "gamma"=w115) -> ("Array"=w117:dbl[])  [unwired: 8 in]
          }
        }
        n31 = for {
          N -> [w81]
          tunnel: w53 -> [w90] mode=indexing
          tunnel: w64 -> [w87]
          shift-right: [w86] -> w63
          shift-left: w62 -> [w85]
          tunnel: [w84] -> w61 mode=indexing
          tunnel: [w83] -> w60 mode=indexing
          i -> [w82]
          n32 = flat-sequence {
            tunnel: w90 -> [w100]
            tunnel: [w101] -> w88
            tunnel: w85 -> [w99]
            tunnel: [w104] -> w89
            tunnel: w88 -> [w104]
            tunnel: w87 -> [w103]
            tunnel: w89 -> [w109]
            tunnel: [w108] -> w86
            tunnel: [w107] -> w84
            tunnel: [w106] -> w83
            frame #0 {
              n33 = call "PLL analyzer -- data source -- V1.vi"("data source action"=data_source_action."set", "Freq in (Hz)"=w100, "PLL data source"=w99) -> ("PLL data source OUT"=w101:T4)  [unwired: 6 in, 2 out]
            }
            frame #1 {
              n34 = Wait Until Next ms Multiple(millisecond multiple=w103) -> ()  [unwired: 1 out]
            }
            frame #2 {
              n35 = call "PLL analyzer -- data source -- V1.vi"("data source action"=data_source_action."get", "PLL data source"=w109) -> ("z out (V)"=w107:cdb, "Freq out (Hz)"=w106:dbl, "PLL data source OUT"=w108:T4)  [unwired: 7 in]
            }
          }
          n36 = case shown="True" "beep!" {
            tunnel: w82 -> [_ w94]
            tunnel: w81 -> [_ w93]
            frame False {
            }
            frame True {
              n37 = Quotient & Remainder(x=w93, y=2) -> (floor(x/y)=w96:i32)  [unwired: 1 out]
              n38 = Equal?(x=w94, y=w96) -> (x = y?=w95:bool)
              n39 = case shown="True" w95 {
                frame False {
                }
                frame True {
                  n40 = call <vilib>:"Beep.vi"("use system alert? (T) - ignored"=FALSE) -> ()  [unwired: 11 in]
                }
              }
            }
          }
          n41 = disable-structure shown="Disabled" {
            disable-tunnel: w82 -> [w91 _]
            frame Disabled {
              n42 = call "MFLI -- publish -- progress.vi"("publisher action"=publisher_action."set", "num"=w91) -> ()  [unwired: 9 in, 1 out]
            }
            frame Enabled {
            }
          }
          "scan progress" <- w82
        }
        n43 = Delete From Array(array=w60, length=1, index=0) -> (array with subset deleted=w57:dbl[])  [unwired: 1 out]
        n44 = Delete From Array(array=w61, length=1, index=0) -> (array with subset deleted=w56:cdb[])  [unwired: 1 out]
        n45 = call "array -- sort 2D array -- Complex.vi"("z In"=w56, "freq IN"=w57) -> ("z out"=w54:cdb[], "freq out"=w55:dbl[])  [unwired: 8 in]
        n46 = flat-sequence {
          tunnel: w54 -> [w119]
          tunnel: w55 -> [w118]
          tunnel: w59 -> [w122]
          tunnel: "New sweep data arrives" ("event data") -> [w121]
          frame #0 {
            n47 = call "MFLI -- publish -- freq scan.vi"("publisher action"=publisher_action."set", "Voltage IN (V)"=w119, "Freq IN (Hz)"=w118) -> ()  [unwired: 7 in, 2 out]
          }
          frame #1 {
            n48 = Generate User Event(user event=w122, event data cluster=w121) -> ()  [unwired: 2 in, 2 out]
          }
        }
      }
    }
  }
  n49 = Create User Event(user event datatype=w41) -> (user event=w40:refnum<user-event>)  [unwired: 1 in, 1 out]
  n50 = register-events(w40) -> (reference out=w42:refnum<event-registration>)  [unwired: 2 in, 1 out]
  n51 = while {
    tunnel: w44 -> [w132]
    tunnel: w29 -> [w130]
    tunnel: w33 -> [w126]
    tunnel: w4 -> [w124]
    tunnel: w5 -> [w123]
    i -> [w127]
    stop <- FALSE stop-if-true
    n52 = Equal To 0?(x=w127) -> (x = 0?=w125:bool)
    n53 = event shown="[0] <calculate>: User Event" {
      selector: w132 -> [_ _]
      dyn-events: _ -> [_ _]
      timeout: 1 -> [_ _]
      tunnel: w130 -> [w140 _]
      tunnel: w126 -> [w137 _]
      tunnel: w125 -> [w136 _]
      tunnel: w124 -> [w135 _]
      tunnel: w123 -> [w133 _]
      event User Event {
        # "all z"
        # "all omega"
        n54 = event-data() -> ("calculate"=w141:string)  [unwired: 1 in]
        n55 = local read "lorentzian"() -> (w134:T6)
        n56 = for {
          N: 1 -> [_]
          tunnel: w141 -> [w149]
          tunnel: w140 -> [w148]
          tunnel: "Save folder" -> [w147]
          tunnel: w137 -> [w146]
          tunnel: w136 -> [w145]
          tunnel: w135 -> [w144]
          tunnel: w134 -> [w143]
          tunnel: w133 -> [w142]
          n57 = case shown="\"Fit\"" w149 {
            tunnel: w148 -> [w160 w183 _ _ _ _]
            tunnel: w147 -> [_ _ w207 w229 _ _]
            tunnel: w146 -> [_ _ _ _ w251 _]
            tunnel: w145 -> [_ _ _ _ _ _]
            tunnel: w144 -> [_ _ _ w230 w250 _]
            tunnel: w143 -> [_ _ _ w228 _ _]
            tunnel: w142 -> [_ _ _ w221 _ _]
            frame "New sweep data arrives" {
              n58 = Generate User Event(user event=w160, event data cluster="Fit" ("event data")) -> (user event out=w151:refnum<user-event>)  [unwired: 2 in, 1 out]
              n59 = case shown="True" "Auto-update sweep window!" {
                tunnel: w151 -> [_ w181]
                frame False {
                }
                frame True {
                  n60 = Generate User Event(user event=w181, event data cluster="Update range" ("event data")) -> ()  [unwired: 2 in, 2 out]
                }
              }
              n61 = call "MFLI -- publish -- freq scan.vi"("publisher action"=publisher_action."get") -> ("Voltage out (V)"=w155:cdb[], "Freq out (Hz)"=w157:dbl[])  [unwired: 9 in]
              n62 = case shown="True" "subtract bgnd !" {
                tunnel: w157 -> [w172 w180]
                tunnel: [w166 w180] -> w156
                tunnel: w155 -> [w168 w179]
                tunnel: [w173 w179] -> w154
                frame True {
                  w165 = 10 ("length")
                  n63 = Delete From Array(array=w172, length=w165, index=0) -> (array with subset deleted=w171:dbl[])  [unwired: 1 out]
                  n64 = Delete From Array(array=w168, length=w165, index=0) -> (array with subset deleted=w167:cdb[])  [unwired: 1 out]
                  n65 = call "linear interp iiii- complex - z-omega.vi"("z"=w167, "omega"=w171) -> ("z out"=w174:cdb[], "omega out"=w166:dbl[], "intercept"=w176:cdb, "slope"=w177:cdb)  [unwired: 5 in, 5 out]
                  n66 = Multiply(x=w166, y=w177) -> (x*y=w178:cdb[])
                  n67 = Add(x=w178, y=w176) -> (x+y=w175:cdb[])
                  n68 = Subtract(x=w174, y=w175) -> (x-y=w173:cdb[])
                }
                frame False {
                }
              }
              n69 = Complex To Re/Im(x + iy=w154) -> (x=w163:dbl[], y=w162:dbl[])
              n70 = Bundle("Freq out (Hz)"=w156, w163) -> (w164:cluster{"Freq out (Hz)":dbl[], dbl[]})  [unwired: 1 in]
              n71 = Bundle("Freq out (Hz)"=w156, w162) -> (w161:cluster{"Freq out (Hz)":dbl[], dbl[]})  [unwired: 1 in]
              n72 = Build Array(w164, w161) -> (→"Plot: circle sweep window":cluster{"Freq out (Hz)":dbl[], dbl[]}[])
            }
            frame "read from disk" {
              n73 = call "file - read-write - list of lines.vi"("read/write control"=file_--_read-write_control."read", "file path"="read file") -> ("list of lines OUT"=w187:string[])  [unwired: 8 in, 1 out]
              n74 = for {
                tunnel: w187 -> [w197] mode=indexing
                tunnel: [w192] -> w188 mode=indexing
                tunnel: [w191] -> w189 mode=indexing
                w193 = 0.0
                n75 = Scan From String(format string="%f%f%f", input string=w197, default 1=w193, default 2=w193, default 3=w193) -> (output 1=w191:dbl, output 2=w195:dbl, output 3=w194:dbl)  [unwired: 2 in, 3 out]
                n76 = Re/Im To Complex(1:w194, 2:w195) -> (0:w192:cdb)
              }
              n77 = flat-sequence {
                tunnel: w183 -> [w201]
                tunnel: [w201] -> w190
                tunnel: w188 -> [w199]
                tunnel: w189 -> [w198]
                tunnel: w190 -> [w203]
                tunnel: "New sweep data arrives" ("event data") -> [w202]
                frame #0 {
                  n78 = call "MFLI -- publish -- freq scan.vi"("publisher action"=publisher_action."set", "Voltage IN (V)"=w199, "Freq IN (Hz)"=w198) -> ()  [unwired: 7 in, 2 out]
                }
                frame #1 {
                  n79 = Generate User Event(user event=w203, event data cluster=w202) -> ()  [unwired: 2 in, 2 out]
                }
              }
            }
            frame "save freq scan" {
              n80 = local read "freqsweep name template"() -> (w209:T2)
              n81 = call "MFLI -- publish -- freq scan.vi"("publisher action"=publisher_action."get") -> ("Voltage out (V)"=w204:cdb[], "Freq out (Hz)"=w205:dbl[])  [unwired: 9 in]
              n82 = call "filename-manage.vi"("filename pattern"=w209, "filename-action"=filename-action."uniquenum", "folder"=w207, "file name"="freq sweep file name") -> ("filename OUT"=w208:string)  [unwired: 7 in]
              n83 = call "KM_appendline -- freq sweep.vi"("freq"=w205, "Vout(V)"=w204, "Save frequency scan"=w207, "read/write control"=KM_file_--_read-write_control."append one line", "name or relative path"=w208) -> ()  [unwired: 15 in]
              n84 = local write "freq sweep file name"(w208) -> ()
            }
            frame "Update range" {
              n85 = call "cursor window logic V3.vi"("cursor window action"=cursor_window_action."read", "cursor window in"=w221) -> ("cursor window out"=w224:T12)  [unwired: 8 in, 1 out]
              n86 = Unbundle By Name(w224) -> ("left"=w223:dbl, "right"=w222:dbl, "window"=w216:dbl)
              n87 = Unbundle By Name(w228) -> ("omega(0)"=w219:dbl, "Gamma"=w226:dbl)
              n88 = Multiply(x=w216, y=3.0 ("lower")) -> (x*y=w217:dbl)
              n89 = Multiply(x=w216, y=0.0003 ("lower")) -> (x*y=w214:dbl)
              n90 = call "Q -- check range -- i -- real.vi"("upper"=w222, "lower"=w223, "number"=w219) -> ("in range?"=w227:bool)  [unwired: 6 in, 2 out]
              n91 = call "Q -- check range -- i -- real.vi"("upper"=w217, "lower"=w214, "number"=w226) -> ("in range?"=w225:bool)  [unwired: 6 in, 2 out]
              n92 = And(x=w227, y=w225) -> (x .and. y?=w220:bool)
              "fit is fine" <- w220
              n93 = case shown="True" w220 {
                tunnel: w226 -> [_ w238]
                tunnel: w219 -> [_ w233]
                tunnel: w230 -> [_ w239]
                tunnel: w229 -> [_ _]
                frame False {
                }
                frame True {
                  (unwired) agregator_--_action."append" ("aggregator action")
                  n94 = Compound Arithmetic op=MULTIPLY("gamma factor", w238, 2.0 ("value")) -> (w236:dbl)
                  n95 = for {
                    N: 1 -> [_]
                    tunnel: "history length" -> [w243]
                    tunnel: w233 -> [w248]
                    shift-right: [w244] -> _
                    shift-left: _ -> [w247]
                    tunnel: [w241] -> w232
                    n96 = call "aggregator - vii - real - atomic.vi"("aggregator action"=agregator_--_action."append", "requested size"=w243, "number"=w248, "state IN"=w247) -> ("state OUT"=w245:T21)  [unwired: 4 in, 3 out]
                    n97 = call "aggregator - vii - real - atomic.vi"("aggregator action"=agregator_--_action."interpolate", "requested size"=w243, "state IN"=w245) -> ("interp average"=w241:dbl, "state OUT"=w244:T21)  [unwired: 5 in, 2 out]
                  }
                  n98 = call "cursor window logic V3.vi"("cursor window action"=cursor_window_action."change cen&win", "window"=w236, "center"=w232, "cursor window in"=w239) -> ()  [unwired: 6 in, 2 out]
                }
              }
            }
            frame "Fit" {
              n99 = case shown="True" "fit!" {
                tunnel: w251 -> [_ w266]
                tunnel: w250 -> [_ w264]
                frame False {
                  (unwired) T6 {"Amplitude"=-1.0311345636926572, "omega(0)"=-1.0311345636926572, "Gamma"=-1.0311345636926572, "phase"=-1.0311345636926572, "Q"=-1.0311345636926572, "Norm  Ampl"=-1.0311345636926572, "z (inf)"=-1.0311345636926572+0.0i, "4corners"={"z (-pi/2)"=-1.0311345636926572+0.5736824521422934i, "z(inf)"=-0.5200164984937075+1.0975277942502903i, "z (pi/2)"=-1.0311345636926572+0.5736824521422934i, "z center"=-0.5136528600391839+0.580046090596817i, "z(0)"=-0.5200164984937075+1.0975277942502903i, "radius"=-1.0311345636926572}} ("pm lorentzian")
                }
                frame True {
                  n100 = call "cursor window logic V3.vi"("cursor window action"=cursor_window_action."read", "cursor window in"=w264) -> ("cursor window out"=w261:T12)  [unwired: 8 in, 1 out]
                  n101 = call "MFLI -- publish -- freq scan.vi"("publisher action"=publisher_action."get") -> ("Voltage out (V)"=w252:cdb[], "Freq out (Hz)"=w253:dbl[])  [unwired: 9 in]
                  n102 = call "acquire cursor window data.vi"("z in"=w252, "omega in"=w253, "cursor window"=w261) -> ("z out"=w262:cdb[], "omega  out"=w263:dbl[])  [unwired: 4 in, 3 out]
                  n103 = call "KM_peak -- find -- pm - V1.vi"("omega in"=w263, "z in"=w262, "parameters: complex fit"="parameters: complex fit", "plots: filter related"=w266, "plot staff ?"="plot staff!", "just guess?"="use fast fit!", "subtract linear BG"=FALSE) -> ("pm lorentzian"=w255:T6)  [unwired: 10 in, 2 out]
                  n104 = local write "lorentzian"(w255) -> ()
                  n105 = Unbundle By Name(w255) -> ("omega(0)"=→"circle frequency (Hz)":dbl, "Gamma"=→"circle gamma (Hz)":dbl, "phase"=→"circle phase (rad)":dbl, "Q"=→"circle Q":dbl)
                  n106 = call "publish -- lorentzian.vi"("publisher action"=publisher_action."set", "lorentzian IN"=w255) -> ()  [unwired: 9 in, 1 out]
                }
              }
            }
            frame "Void", Default {
            }
          }
        }
      }
      event Timeout {
        n107 = event-data() -> ()  [unwired: 1 in, 2 out]
      }
    }
    n108 = Wait (ms)(milliseconds to wait=u32 0) -> ()  [unwired: 1 out]
  }
  n109 = while {
    tunnel: w42 -> [w277]
    tunnel: w29 -> [w275]
    tunnel: w4 -> [w274]
    tunnel: w5 -> [w271]
    stop <- FALSE stop-if-true
    n110 = local read "lorentzian"() -> (w273:T6)
    n111 = Wait (ms)(milliseconds to wait=u32 0) -> ()  [unwired: 1 out]
    n112 = event shown="[4] \"scale gauge: Plot: complex plane - filter\": Value Change" {
      selector: w277 -> [_ _ _ _ _ _ _ _]
      dyn-events: _ -> [_ _ _ _ _ _ _ _]
      timeout: _ -> [_ _ _ _ _ _ _ _]
      tunnel: w275 -> [_ w278 w298 _ _ w320 _ w334]
      tunnel: w274 -> [_ w281 _ _ _ _ w322 w330]
      tunnel: w273 -> [_ _ _ w308 w317 _ _ _]
      tunnel: w271 -> [_ w279 _ _ _ _ _ w329]
      tunnel: [_ _ _ _ _ "read from disk :l" _ _] -> _
      event Timeout {
        n113 = event-data() -> ()  [unwired: 1 in, 2 out]
      }
      event "Plot: circle sweep window": Cursor Move {
        n114 = event-data() -> ("CursIdx"=w280:i32)  [unwired: 1 in, 8 out]
        n115 = case shown="0..2" w280 {
          selector: w280 -> [w291 w295]
          tunnel: w281 -> [w293 _]
          tunnel: w279 -> [_ w294]
          tunnel: w278 -> [w289 _]
          frame 0..2 {
            w288 = "Fit"  # event data
            n116 = call "cursor window logic V3.vi"("CursIdx"=w291, "cursor window action"=cursor_window_action."cursor moves", "cursor window in"=w293) -> ("cursor window out"=w290:T12)  [unwired: 7 in, 1 out]
            n117 = Generate User Event(user event=w289, event data cluster=w288) -> ()  [unwired: 2 in, 2 out]
            n118 = Unbundle By Name(w290) -> ("left"=w285:dbl, "right"=w284:dbl, "center"=w283:dbl, "window"=w282:dbl)
            n119 = Bundle By Name(cluster=T3 {"cen (Hz)"=-0.35260838541595674, "win (Hz)"=17.234446484426172, "left (Hz)"=-8.969831627629043, "right (Hz)"=8.26461485679713} ("win"), "left (Hz)"=w285, "right (Hz)"=w284, "cen (Hz)"=w283, "win (Hz)"=w282) -> (w286:T3)
            n120 = local write "win"(w286) -> ()
          }
          frame 3..5, Default {
            n121 = call "cursor window logic V3.vi"("CursIdx"=w295, "cursor window action"=cursor_window_action."cursor moves", "cursor window in"=w294) -> ()  [unwired: 7 in, 2 out]
          }
        }
      }
      event "Plot: circle sweep window": Cursor Release {
        n122 = event-data() -> ("CursIdx"=w297:i32)  [unwired: 1 in, 8 out]
        n123 = case shown="3, Default" w297 {
          tunnel: w298 -> [_ w299]
          frame 3, Default {
          }
          frame 0..2 {
            w300 = "Fit"  # event data
            n124 = Generate User Event(user event=w299, event data cluster=w300) -> ()  [unwired: 2 in, 2 out]
          }
        }
      }
      event "scale gauge: Plot: complex plane": Value Change {
        n125 = event-data() -> ("NewVal"=w302:dbl)  [unwired: 1 in, 5 out]
        n126 = Unbundle By Name(w308) -> ("4corners.z center"=w309:cdb)
        n127 = control-ref of="Plot: complex plane"() -> (w307:refnum<vi>)
        n128 = Complex To Re/Im(x + iy=w309) -> (x=w304:dbl, y=w303:dbl)
        n129 = Bundle By Name(cluster=T22 {"window y"=0.0021014740628288917, "center x"=44850.89441339177, "center y"=2.5658109925320947, "window x"=17480.201988350764} ("window IN"), "window x"=w302, "window y"=w302, "center x"=w304, "center y"=w303) -> (w301:T22)
        n130 = call "replace cursor - plot ref - V2.vi"("Plot ref in"=w307, "window IN"=w301, "cursor action"=cursor_action."zoom to win") -> ()  [unwired: 14 in, 3 out]
      }
      event "scale gauge: Plot: complex plane - filter": Value Change {
        n131 = event-data() -> ("NewVal"=w312:dbl)  [unwired: 1 in, 5 out]
        n132 = Unbundle By Name(w317) -> ("4corners.z center"=w318:cdb)
        n133 = control-ref of="Plot: complex plane - filter"() -> (w313:refnum<vi>)
        n134 = Complex To Re/Im(x + iy=w318) -> (x=w311:dbl, y=w310:dbl)
        n135 = Bundle By Name(cluster=T22 {"window y"=0.0021014740628288917, "center x"=44850.89441339177, "center y"=2.5658109925320947, "window x"=17480.201988350764} ("window IN"), "window x"=w312, "window y"=w312, "center x"=w311, "center y"=w310) -> (w314:T22)
        n136 = call "replace cursor - plot ref - V2.vi"("Plot ref in"=w313, "window IN"=w314, "cursor action"=cursor_action."zoom to win") -> ()  [unwired: 14 in, 3 out]
      }
      event "read from disk :l": Value Change {
        n137 = event-data() -> ()  [unwired: 1 in, 6 out]
        n138 = Generate User Event(user event=w320, event data cluster="read from disk" ("event data")) -> ()  [unwired: 2 in, 2 out]
      }
      event Value Change {
        n139 = event-data() -> ("NewVal"=w325:T3)  [unwired: 1 in, 5 out]
        n140 = Unbundle By Name(w325) -> ("cen (Hz)"=w323:dbl, "win (Hz)"=w324:dbl)
        n141 = call "cursor window logic V3.vi"("cursor window action"=cursor_window_action."change center", "center"=w323, "cursor window in"=w322) -> ("cursor window out"=w326:refnum<vi>)  [unwired: 7 in, 1 out]
        n142 = call "cursor window logic V3.vi"("cursor window action"=cursor_window_action."change window", "window"=w324, "cursor window in"=w326) -> ()  [unwired: 7 in, 2 out]
      }
      event Key Down {
        n143 = event-data() -> ("Char"=w332:i16, "VKey"=w335:T24)  [unwired: 1 in]
        n144 = Build Array(w332) -> (w333:i16[])
        n145 = Byte Array To String(unsigned byte array=w333) -> (string=w331:string)
        n146 = case shown="\"ASCII\", Default" w335 {
          selector: w335 -> [_ _ _ _ w387]
          tunnel: w332 -> [_ _ _ _ _]
          tunnel: w334 -> [w339 _ _ _ w386]
          tunnel: w331 -> [w338 _ _ _ _]
          tunnel: w330 -> [w337 _ _ _ w383]
          tunnel: w329 -> [w336 _ _ _ _]
          frame "ASCII", Default {
            n147 = case shown="\"t\"" w338 {
              selector: w338 -> [_ _ _ _ _ _ w351 _ _ _]
              tunnel: w339 -> [_ _ w342 w344 w346 _ _ _ _ _]
              tunnel: w337 -> [_ w340 _ _ _ w348 w352 w359 w366 w375]
              tunnel: w336 -> [_ _ _ _ _ _ _ w357 _ _]
              frame "0", Default {
              }
              frame "a" {
                n148 = call "cursor window logic V3.vi"("cursor window action"=cursor_window_action."zoom to all data", "cursor window in"=w340) -> ()  [unwired: 8 in, 2 out]
              }
              frame "s" {
                n149 = Generate User Event(user event=w342, event data cluster="save freq scan" ("event data")) -> ()  [unwired: 2 in, 2 out]
              }
              frame "l" {
                n150 = Generate User Event(user event=w344, event data cluster="read from disk" ("event data")) -> ()  [unwired: 2 in, 2 out]
              }
              frame "p" {
                n151 = Generate User Event(user event=w346, event data cluster="New sweep data arrives" ("event data")) -> ()  [unwired: 2 in, 2 out]
              }
              frame "?" {
                # "?"
                n152 = call "cursor window logic V3.vi"("cursor window action"=cursor_window_action."zoom X", "cursor window in"=w348) -> ()  [unwired: 8 in, 2 out]
              }
              frame "+", "-", "<", ">" {
                # "?"
                n153 = case shown="\"+\", Default" w351 {
                  tunnel: [cursor_window_action."slide right" ("cursor window action") cursor_window_action."slide left" ("cursor window action") cursor_window_action."zoom in" ("cursor window action") cursor_window_action."zoom out" ("cursor window action")] -> w350
                  frame ">" {
                  }
                  frame "<" {
                  }
                  frame "+", Default {
                  }
                  frame "-" {
                  }
                }
                n154 = call "cursor window logic V3.vi"("cursor window action"=w350, "cursor window in"=w352) -> ()  [unwired: 8 in, 2 out]
              }
              frame "c" {
                n155 = call "cursor window logic V3.vi"("cursor window action"=cursor_window_action."check", "cursor window in"=w357) -> ()  [unwired: 8 in, 2 out]
                n156 = call "cursor window logic V3.vi"("cursor window action"=cursor_window_action."check", "cursor window in"=w359) -> ()  [unwired: 8 in, 2 out]
              }
              frame "t" {
                n157 = local read "Auto-update sweep window!"() -> (w365:bool)
                n158 = Not(x=w365) -> (.not. x?=w364:bool)
                n159 = Select(t=cursor_window_action."color--green" ("cursor window action"), s=w364, f=cursor_window_action."color--red" ("cursor window action")) -> (s? t:f=w361:T14)
                n160 = local write "Auto-update sweep window!"(w364) -> ()
                n161 = call "cursor window logic V3.vi"("cursor window action"=w361, "cursor window in"=w366) -> ()  [unwired: 8 in, 2 out]
              }
              frame "r" {
                n162 = local read "Auto-update sweep window!"() -> (w370:bool)
                n163 = local read "sweep! :r"() -> (w371:bool)
                n164 = Not(x=w371) -> (.not. x?=w374:bool)
                n165 = Select(t=cursor_window_action."color--green" ("cursor window action"), s=w370, f=cursor_window_action."color--red" ("cursor window action")) -> (s? t:f=w367:T14)
                n166 = Select(t=w367, s=w374, f=cursor_window_action."color--yellow" ("cursor window action")) -> (s? t:f=w372:T14)
                n167 = local write "sweep! :r"(w374) -> ()
                n168 = call "cursor window logic V3.vi"("cursor window action"=w372, "cursor window in"=w375) -> ()  [unwired: 8 in, 2 out]
              }
            }
          }
          frame "Escape" {
          }
          frame "PageUp" {
          }
          frame "PageDown" {
          }
          frame "Up".."Right" {
            w376 = "Fit"  # event data
            n169 = case shown="\"Left\"" w387 {
              tunnel: [cursor_window_action."move right" ("cursor window action") cursor_window_action."move left" ("cursor window action") cursor_window_action."broaden" ("cursor window action") cursor_window_action."shrink" ("cursor window action")] -> w385
              frame "Right", Default {
              }
              frame "Left" {
              }
              frame "Up" {
              }
              frame "Down" {
              }
            }
            n170 = call "cursor window logic V3.vi"("cursor window action"=w385, "cursor window in"=w383) -> ("cursor window out"=w384:T12)  [unwired: 8 in, 1 out]
            n171 = Unbundle By Name(w384) -> ("left"=w380:dbl, "right"=w379:dbl, "center"=w378:dbl, "window"=w377:dbl)
            n172 = Bundle By Name(cluster=T3 {"cen (Hz)"=-0.35260838541595674, "win (Hz)"=17.234446484426172, "left (Hz)"=-8.969831627629043, "right (Hz)"=8.26461485679713} ("win"), "left (Hz)"=w380, "right (Hz)"=w379, "cen (Hz)"=w378, "win (Hz)"=w377) -> (w382:T3)
            n173 = Generate User Event(user event=w386, event data cluster=w376) -> ()  [unwired: 2 in, 2 out]
            n174 = local write "win"(w382) -> ()
          }
        }
      }
    }
  }
